vi "ISX3_Cmd_GetSetupLoad.vi"(1 "Setup Slot":u8=1 min=1 step=1) -> (0 "get Setup Load Cmd":u8[](array[numeric]))   [LabVIEW 2012, in "Sciospec ISX3 Impedance Analyzer.lvlib"]
uses:
  Sciospec ISX3 Impedance Analyzer.lvlib
panel:
  # "This VI generates the command to load a setup to the device.\nThere are 255 available slots."
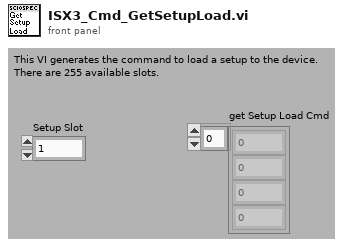
[diagram p1: front panel]
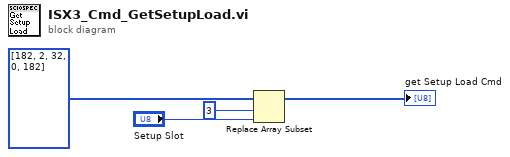
[diagram p0: block diagram]
diagram:
  n1 = Replace Array Subset(array=u8[] [182, 2, 32, 0, 182], new element="Setup Slot", index=3) -> (→"get Setup Load Cmd":u8[])
